vi "Write Page Data.vi"(0 "Byte Stream File in":refnum<file>, 1 "Details":T4={"ImageDescription"="", "XResolution"=0.0, "YResolution"=0.0, "ResolutionUnit"=enum."Inch", "PhotometricInterpretation"=0, "Compression"=enum."None", "PageName"="", "DocumentName"=""} {"PhotometricInterpretation" items=["PHOTOMETRIC_MINISWHITE"=0, "PHOTOMETRIC_MINISBLACK"=1, "PHOTOMETRIC_RGB"=2, "PHOTOMETRIC_PALETTE"=3, "PHOTOMETRIC_MASK"=4, "PHOTOMETRIC_SEPARATED"=5, "PHOTOMETRIC_YCBCR"=6, "PHOTOMETRIC_CIELAB"=8, "PHOTOMETRIC_ICCLAB"=9, "PHOTOMETRIC_ITULAB"=10, "PHOTOMETRIC_LOGL"=32844, "PHOTOMETRIC_LOGLUV"=32845, "CFA"=32803, "LinearRaw"=34892, "DEPTH"=51177]}, 2 "Additional Named Tags":cluster{"name":string, "Variant":variant}[](array[cluster]), 3 "Image":variant, 5 "Offset":i64=8, 7 "IFD Offset Position":i64 format="%x", 9 "byte order (0:big-endian, network order)":T5(ring)=enum."little-endian", 11 "error in (no error)":errorcluster, 12 "Settings":T3={"zlib compression level"=-1, "Max Strip bytes"=8192, "JPEG Quality (85)"=85}, 13 "Additional Tags":T2(array[cluster])) -> (4 "Byte Stream File out":refnum<file>, 6 "Next Offset":i64 format="%x", 8 "Next IFD Offset Position":i64 format="%x", 15 "error out":errorcluster)   [LabVIEW 2020, in "LV Tiff.lvlib"]
uses:
  LV Tiff.lvlib
  Tiff Page Details.ctl
  Page Writer Settings.ctl
  Tiff Data Type.ctl
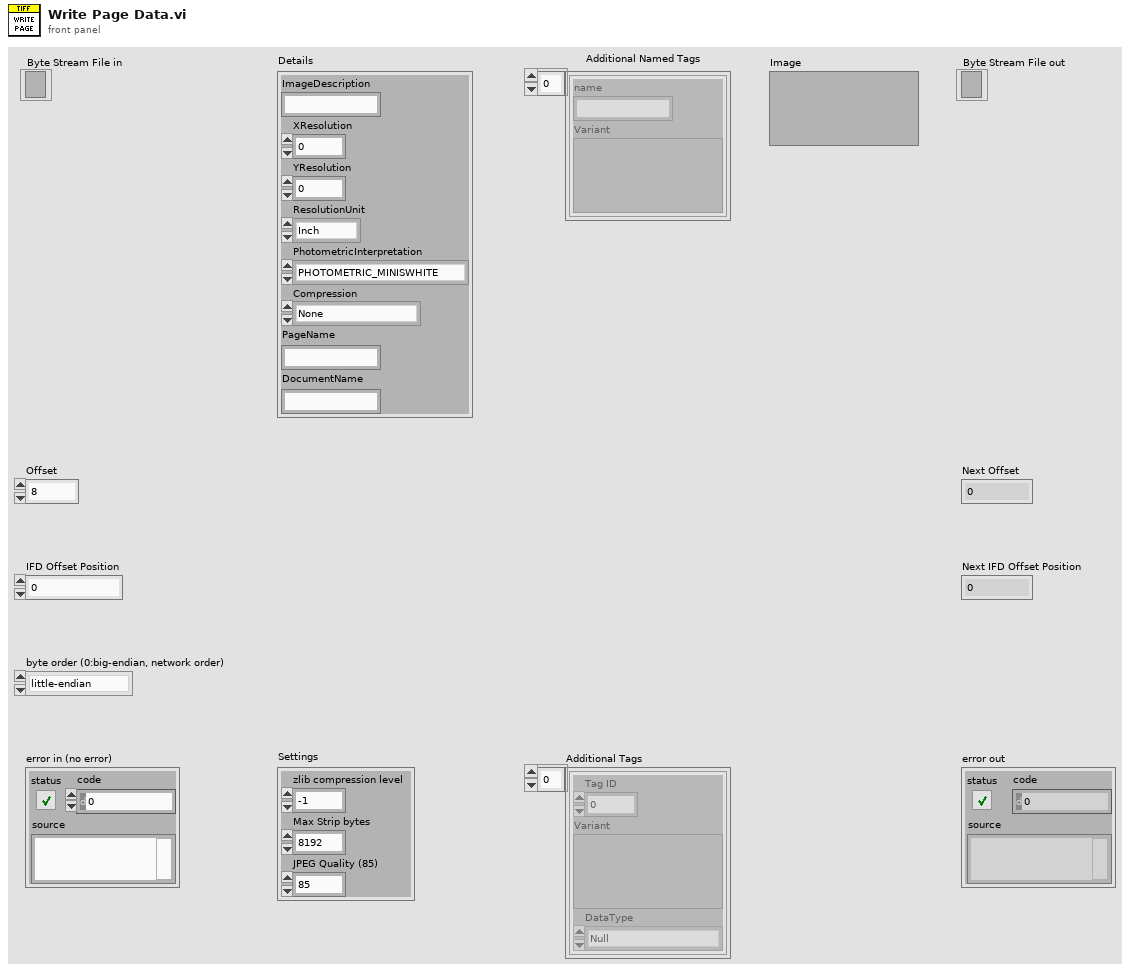
[diagram p1: front panel]
types:
  T1 = typedef "LV Tiff.lvlib/Tiff Data Type.ctl" = enum16{"Null", "BYTE", "ASCII", "SHORT", "LONG", "RATIONAL", "SBYTE", "UNDEFINE", "SSHORT", "SLONG", "SRATIONAL", "FLOAT", "DOUBLE"}
  T2 = cluster{"Tag ID":u32, "Variant":variant, "DataType":T1}[]
  T3 = typedef "LV Tiff.lvlib/Page Writer Settings.ctl" = cluster{"zlib compression level":i32, "Max Strip bytes":u32, "JPEG Quality (85)":i32}
  T4 = typedef "LV Tiff.lvlib/Tiff Page Details.ctl" = cluster{"ImageDescription":string, "XResolution":dbl, "YResolution":dbl, "ResolutionUnit":enum16{"None", "Inch", "Centimeter"}, "PhotometricInterpretation":u16, "Compression":enum16{"None", "Deflate", "JPEG"}, "PageName":string, "DocumentName":string}
  T5 = enum16{"big-endian, network order", "native, host order", "little-endian"}
  T6 = typedef "LV Tiff.lvlib/Baseline Tags 1.ctl" = cluster{"NewSubFileType":u32, "ImageWidth":u32, "ImageHeight":u32, "BitsPerSample":u16, "Compression":u16, "PhotometricInterpretation":u16, "StripOffsets":u32[], "SamplesPerPixel":u16, "RowsPerStrip":u32, "StripByteCounts":u32[], "ResolutionUnit":u16, "SampleFormat":u16}
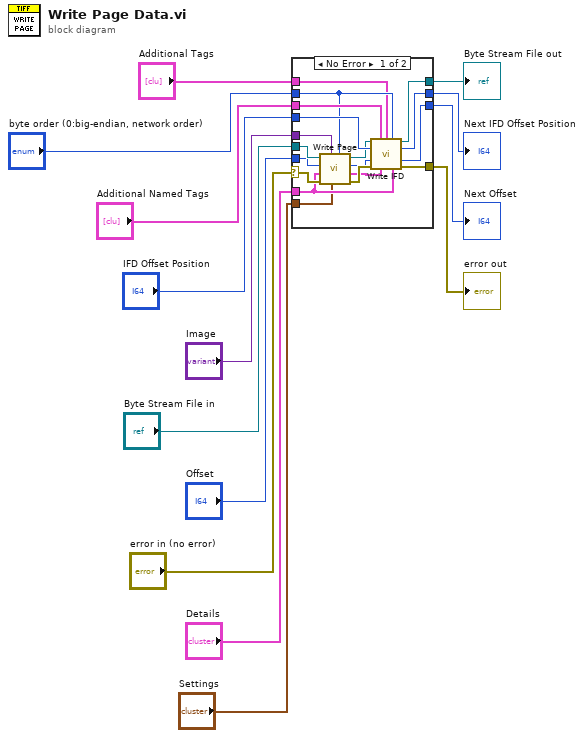
[diagram p0: block diagram]
diagram:
  n1 = case shown="No Error" "error in (no error)" {
    selector: "error in (no error)" -> [w26 w33]
    tunnel: "Offset" -> [w21 _]
    tunnel: "Byte Stream File in" -> [w24 w34]
    tunnel: "Image" -> [w19 _]
    tunnel: "byte order (0:big-endian, network order)" -> [w22 _]
    tunnel: "IFD Offset Position" -> [w32 _]
    tunnel: [w31 w33] -> w8
    tunnel: [w30 _] -> w7
    tunnel: [w29 _] -> w6
    tunnel: [w28 w34] -> w5
    tunnel: "Details" -> [w17 _]
    tunnel: "Additional Named Tags" -> [w27 _]
    tunnel: "Settings" -> [w16 _]
    tunnel: "Additional Tags" -> [w15 _]
    frame No Error {
      n2 = call "Write Page.vi"("byte order (0:big-endian, network order)"=w22, "Settings"=w16, "Image Data"=w19, "error in (no error)"=w26, "Details"=w17, "Offset"=w21, "Byte Stream File in"=w24) -> ("error out"=w25:errorcluster, "IFD Baseline"=w18:T6, "offset (in bytes)"=w20:i64, "Byte Stream File out"=w23:refnum<file>)  [unwired: 1 in]
      n3 = call "Write IFD.vi"("Byte Stream File in"=w23, "Additional Named Tags"=w27, "Additional Tags"=w15, "byte order (0:big-endian, network order)"=w22, "IFD Offset Position"=w32, "Offset"=w20, "error in"=w25, "IFD Baseline"=w18, "Details"=w17) -> ("refnum out"=w28:refnum<file>, "Next IFD Offset Position"=w29:i64, "Next Offset"=w30:i64, "error out"=w31:errorcluster)  [unwired: 3 in]
    }
    frame Error {
    }
  }
  "error out" <- w8
  "Byte Stream File out" <- w5
  "Next Offset" <- w7
  "Next IFD Offset Position" <- w6
